vi "TestConnection.vi"(2 "Python path":path, 3 "Python version":string) -> (0 "error out":errorcluster, 1 "success?":bool)   [LabVIEW 2025]
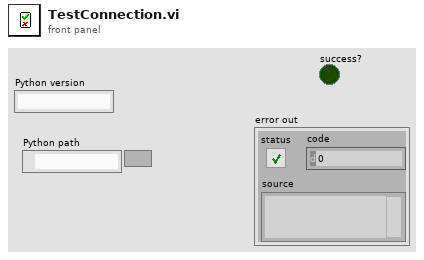
[diagram p1: front panel]
types:
  T1 = cluster{"Python version":string, "Python path":string}
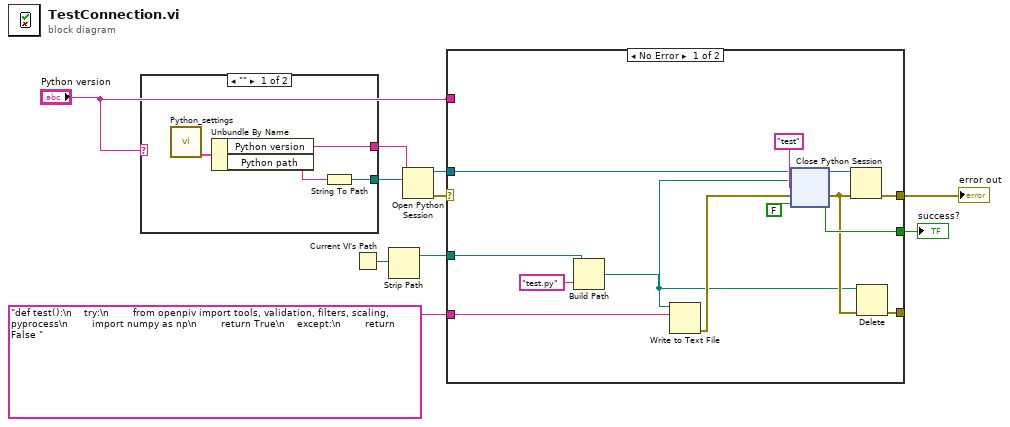
[diagram p0: block diagram]
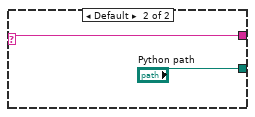
[diagram p2: hidden frame]
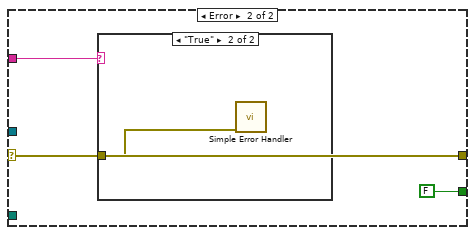
[diagram p3: hidden frame]
diagram:
  n1 = case shown="\"\"" "Python version" {
    selector: "Python version" -> [_ w15]
    tunnel: [w11 "Python path"] -> w8
    tunnel: [w12 w15] -> w6
    frame "" {
      n2 = call "Python_settings.vi"() -> ("settings read"=w13:T1)  [unwired: 5 in]
      n3 = Unbundle By Name(w13) -> ("Python version"=w12:string, "Python path"=w14:string)
      n4 = String To Path(string=w14) -> (path=w11:path)
    }
    frame Default {
    }
  }
  n5 = Current VI's Path() -> (path=w3:path)
  n6 = Strip Path(path=w3) -> (stripped path=w2:path)  [unwired: 1 out]
  n7 = Open Python Session(python version=w6, python path=w8) -> (session out=w10:refnum<k35>, error out=w9:errorcluster)  [unwired: 1 in]
  n8 = case shown="No Error" w9 {
    selector: w9 -> [_ w31]
    tunnel: w10 -> [w27 _]
    tunnel: [w23 FALSE] -> w7
    tunnel: [w22 w31] -> w5
    tunnel: "def test():\n    try:\n        from openpiv import tools, validation, filters, scaling, pyprocess\n        import numpy as np\n        return True\n    except:\n        return False " ("text") -> [w21 _]
    tunnel: w2 -> [w20 _]
    tunnel: "Python version" -> [_ w30]
    tunnel: [w18 _] -> _
    frame No Error {
      n9 = Build Path(base path=w20, name or relative path="test.py" ("Python version")) -> (appended path=w17:path)
      n10 = Write to Text File(file (use dialog)=w17, text=w21) -> (error out=w25:errorcluster)  [unwired: 2 in, 2 out]
      n11 = node(w27, w17, "test" ("function name"), w25, FALSE) -> (w24:refnum<k35>, w19:errorcluster, w23:bool)  [unwired: 2 out]
      n12 = Close Python Session(session in=w24, error in=w19) -> (11:w22:errorcluster)
      n13 = Delete(path (use dialog)=w17, error in=w19) -> (error out=w18:errorcluster)  [unwired: 3 in, 2 out]
    }
    frame Error {
      n14 = case shown="\"True\"" w30 {
        tunnel: w31 -> [_ w33]
        frame "False", Default {
        }
        frame "True" {
          n15 = call <vilib>:"Simple Error Handler.vi"("error in (no error)"=w33) -> ()  [unwired: 4 in, 5 out]
        }
      }
    }
  }
  "success?" <- w7
  "error out" <- w5
